vi "Force Channel.vi"(6 "Force Data":u8[](array[numeric]) format="%.0x", 7 "Channel Array in":refnum<class "CIFChannels.lvclass">[](array[class]), 8 "error in (no error)":errorcluster, 9 "Force Active":bool, 10 "Channel Name":string, 11 "CIFChannelMng in":refnum<class "CIFChannelMng.lvclass">) -> (0 "error out":errorcluster, 2 "Update OOB":bool=TRUE, 3 "CIFChannelMng out":refnum<class "CIFChannelMng.lvclass">, 5 "Channel Array out":refnum<class "CIFChannels.lvclass">[](array[class]))   [LabVIEW 2021, in "CIFChannelMng.lvclass"]
uses:
  CIFChannelMng.lvclass
  CIFChannelMng.lvclass/CIFChannelMng.ctl
  <vilib>/CIF Foundation/CIF Channels Core/CIFChannels/CIFChannels.lvclass
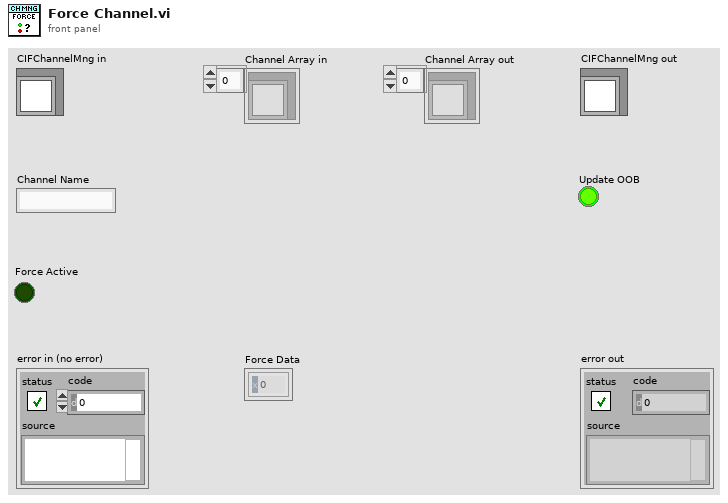
[diagram p1: front panel]
types:
  T1 = typedef "CIFChannelMng.lvclass/Channel List for OOB.ctl" = cluster{"Name":string, "Direction":T2, "Type":string, "Connected?":bool, "Connected Name":string, "Custom Config Data":u8[], "Forced?":bool, "Pattern":T3}
  T2 = typedef "CIFChannels.lvclass/Direction.ctl" = enum16{"Publisher", "Subscriber"}
  T3 = typedef "ChannelCommon.lvlib/Channel Pattern.ctl" = enum16{"Unknown", "Tag", "FIFO", "MultiFIFO", "BackpressureFIFO"}
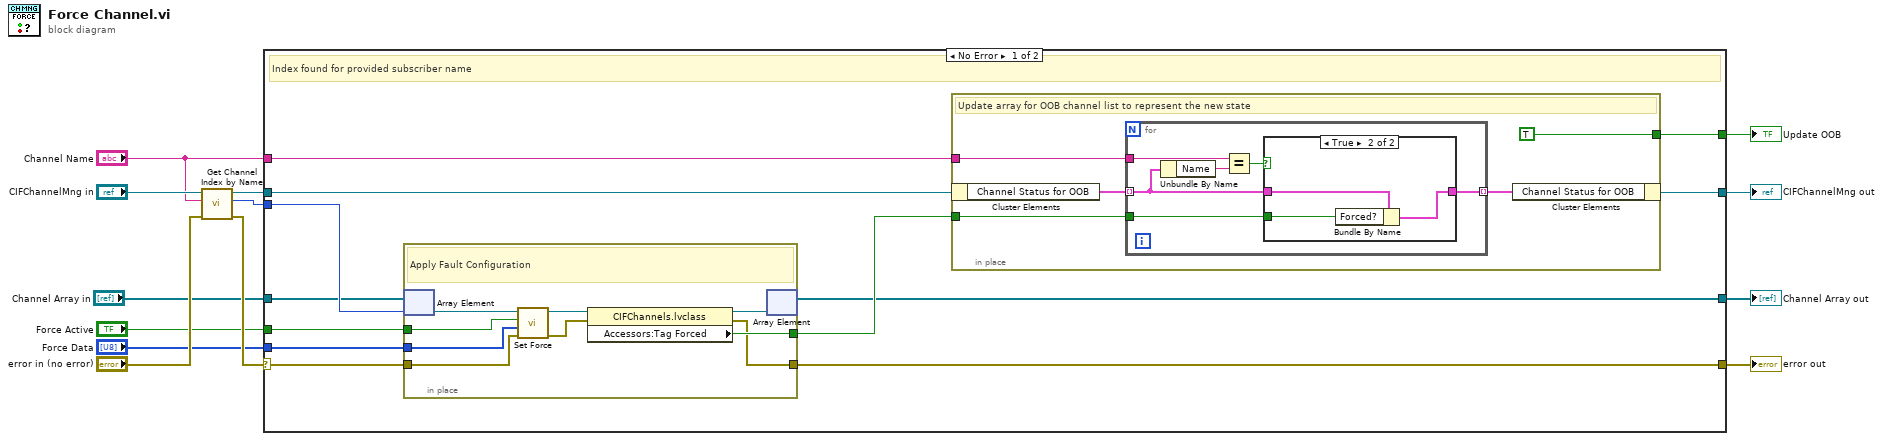
[diagram p0: block diagram]
diagram:
  n1 = call "Get Channel Index by Name.vi"("error in (no error)"="error in (no error)", "Channel Name"="Channel Name", "CIFChannelMng in"="CIFChannelMng in") -> ("error out"=w13:errorcluster, "Channel Index"=w12:i32, "CIFChannelMng out"=w11:refnum<class "CIFChannelMng.lvclass">)  [unwired: 6 in]
  n2 = case shown="No Error" w13 {
    selector: w13 -> [w23 w52]
    tunnel: "Force Data" -> [w25 _]
    tunnel: w11 -> [w14 w51]
    tunnel: w12 -> [w24 _]
    tunnel: "Channel Name" -> [w21 _]
    tunnel: [w20 w51] -> w2
    tunnel: [w19 w52] -> w4
    tunnel: "Force Active" -> [w18 _]
    tunnel: [w17 _] -> w1
    tunnel: "Channel Array in" -> [w16 w50]
    tunnel: [w15 w50] -> w3
    frame No Error {
      # "Index found for provided subscriber name"
      n3 = in-place {
        in-place-border: w25 -> [w34]
        in-place-border: [w27] -> w22
        in-place-border: w23 -> [w32]
        in-place-border: [w26] -> w19
        in-place-border: w18 -> [w31]
        # "Apply Fault Configuration"
        n4 = in-place-array #1(w16, w24) -> (w33:refnum<class "CIFChannels.lvclass">)
        n5 = call <vilib>:"Set Force.vi"("error in (no error)"=w32, "Force Data"=w34, "Force Active"=w31, "CIFChannels in"=w33) -> ("error out"=w28:errorcluster, "CIFChannels out"=w30:refnum<class "CIFChannels.lvclass">)  [unwired: 6 in]
        n6 = property class="CIFChannels.lvclass"(reference=w30, error in=w28) -> (reference out=w29:refnum<class "CIFChannels.lvclass">, error out=w26:errorcluster, "Accessors:Tag Forced"=w27:bool)
        n7 = in-place-array #1(w29) -> (w15:refnum<class "CIFChannels.lvclass">[])  [unwired: 1 out]
      }
      n8 = in-place {
        in-place-border: w22 -> [w36]
        in-place-border: w21 -> [w37]
        in-place-border: [TRUE ("Update OOB")] -> w17
        # "Update array for OOB channel list to represent the new state"
        n9 = in-place-cluster #2(w14) -> ("Channel Status for OOB"=w39:T1[])
        n10 = for {
          tunnel: w39 -> [w44] mode=indexing
          tunnel: w36 -> [w43]
          tunnel: [w42] -> w38 mode=indexing
          tunnel: w37 -> [w40]
          n11 = Unbundle By Name(w44) -> ("Name"=w45:string)
          n12 = Equal?(x=w40, y=w45) -> (x = y?=w41:bool)
          n13 = case shown="True" w41 {
            tunnel: w44 -> [w46 w49]
            tunnel: w43 -> [_ w48]
            tunnel: [w46 w47] -> w42
            frame False {
            }
            frame True {
              n14 = Bundle By Name(cluster=w49, "Forced?"=w48) -> (w47:T1)
            }
          }
        }
        n15 = in-place-cluster #2("Channel Status for OOB"=w38) -> (w20:refnum<class "CIFChannelMng.lvclass">)
      }
    }
    frame Error {
      # "Index by name created error"
    }
  }
  "error out" <- w4
  "CIFChannelMng out" <- w2
  "Update OOB" <- w1
  "Channel Array out" <- w3
